vi "LINX - WS2812 Strip Controller.vi"() -> ()   [LabVIEW 2020]
doc: "Control the RGB colors of a WS2812 light strip using configurable sine, square, triangle and sawtooth waveforms for red, green and blue."
uses:
  vi.lib/MakerHub/LINX/Public/Utilities/Open Serial.vi
  vi.lib/MakerHub/LINX/Public/Sensors/Lights/WS2812/Write N LEDs.vi
  vi.lib/MakerHub/LINX/LMH-LINX.lvlib
  vi.lib/MakerHub/LINX/Public/Sensors/Lights/WS2812/WS2812.lvlib
panel:
  in  "Blue Duty Cycle":dbl=1.0 caption="Phase" min=0.0 max=100.0
  in  "Green Duty Cycle":dbl=1.0 caption="Phase" min=0.0 max=50.0
  in  "Red Duty Cycle":dbl=1.0 caption="Phase" min=0.0 max=100.0
  in  "Blue Waveform":enum16{"Sine", "Square", "Triangle", "Sawtooth"}(ring)
  in  "Green Waveform":enum16{"Sine", "Square", "Triangle", "Sawtooth"}(ring)
  in  "Red Waveform":enum16{"Sine", "Square", "Triangle", "Sawtooth"}(ring)
  in  "Blue Intensity Multiplier":dbl=1.0 caption="Phase" min=0.0 max=1.0
  in  "Green Intensity Multiplier":dbl=1.0 caption="Phase" min=0.0 max=1.0
  in  "Red Intensity Multiplier":dbl=1.0 caption="Phase" min=0.0 max=1.0
  in  "Blue Phase Multiplier":dbl=10.0 caption="Phase"
  in  "Blue Phase Offset":dbl=10.0 caption="Phase"
  in  "Green Phase Multiplier":dbl=10.0 caption="Phase"
  in  "Green Phase Offset":dbl=10.0 caption="Phase"
  in  "Red Phase Offset":dbl=10.0 caption="Phase"
  in  "Red Phase Multiplier":dbl=10.0 caption="Phase"
  out "RGB Values":dynamicdata(graph)
  in  "Stop Button":bool
  in  "Number of LEDs":u16=30
  in  "Data Channel":u8=11
  in  "Serial Port":refnum<visa-resource-name>="COM6"
  # "WS2812 Write N LEDs Example\n\nThis example demonstrates how to set the color of a range of WS2812 LEDs.\n\nInstructions\n1. Select the COM Port associated with the LINX Device.\n2. Select the Data Channel and Number of LEDs.\n3. Click the Run Arrow.\n4. Select the index of the first LED to set.\n5. The number values in the color array determines how many LEDs will be set, starting with the LED at the LED Start Index."
  # "LINX Device Settings"
  # "WS2812 Settings"
  # "Duty Cycle\n(Square Wave)"
  # "Intensity (0-1)"
  # "Phase Multiplier"
  # "Phase Offset"
  # "Waveform"
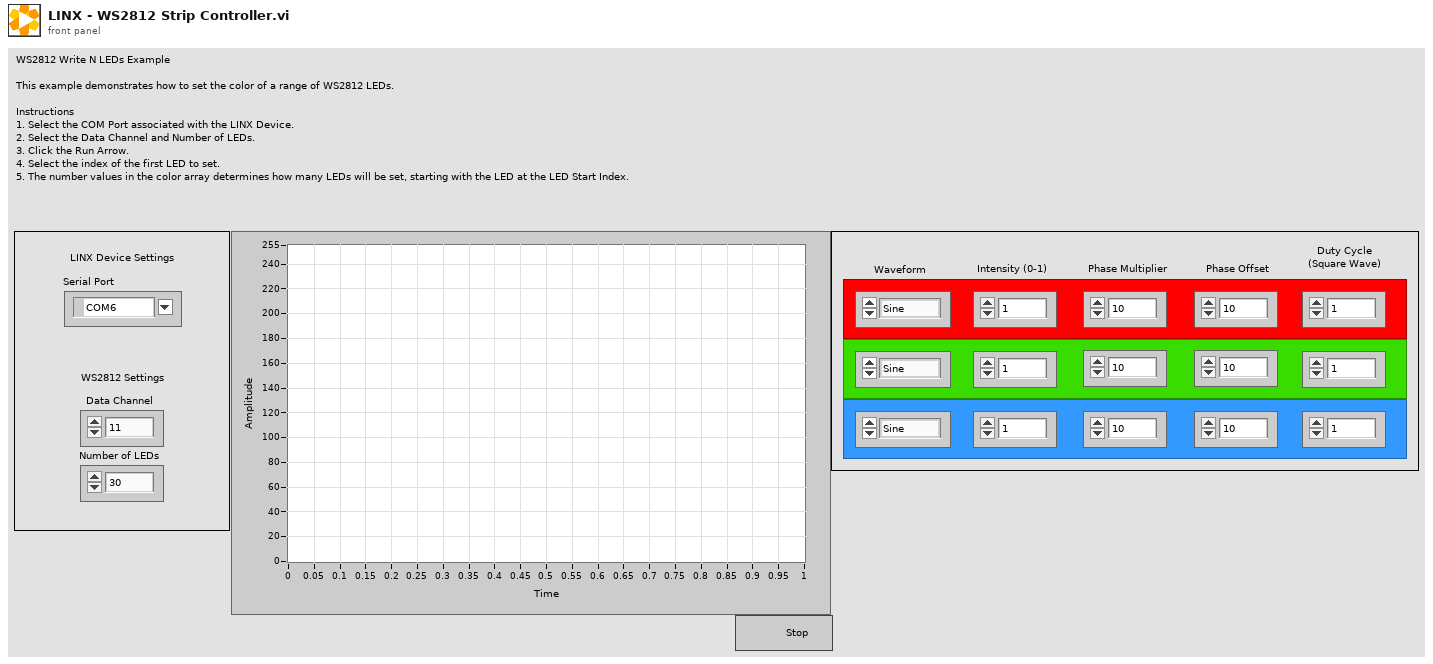
[diagram p1: front panel]
types:
  T1 = typedef "LMH-LINX.lvlib/LINX Ref.ctl" = cluster{"IO":T2, "Interface":T3, "LINX Device Config":T4}
  T2 = typedef "LMH-LINX.lvlib/Platform.ctl" = enum16{"Remote", "Local"}
  T3 = typedef "LMH-LINX.lvlib/Interface.ctl" = enum16{"Serial", "TCP"}
  T4 = typedef "Device.lvlib/LINX Device Config.ctl" = cluster{"Interface":T3, "COM Port":refnum<visa-resource-name>, "TCP Configuration":T5, "Device Family":u8, "Device ID":u8, "Device Name":string, "TCP Ref":refnum<k5>, "Channels":T6}
  T5 = typedef "Device.lvlib/TCP Config.ctl" = cluster{"IP Address":string, "Port":u16}
  T6 = typedef "LMH-LINX.lvlib/Channels.ctl" = cluster{"DI":u8[], "DO":u8[], "AI":u8[], "AO":u8[], "PWM":u8[], "QE":u8[], "UART":u8[], "I2C 2":u8[], "SPI":u8[], "CAN":u8[], "Servo":u8[], "AI Ref (V)":dbl, "AI Resolution (Bits)":u8, "AO Ref (V)":dbl, "AO Resolution (Bits)":u8}
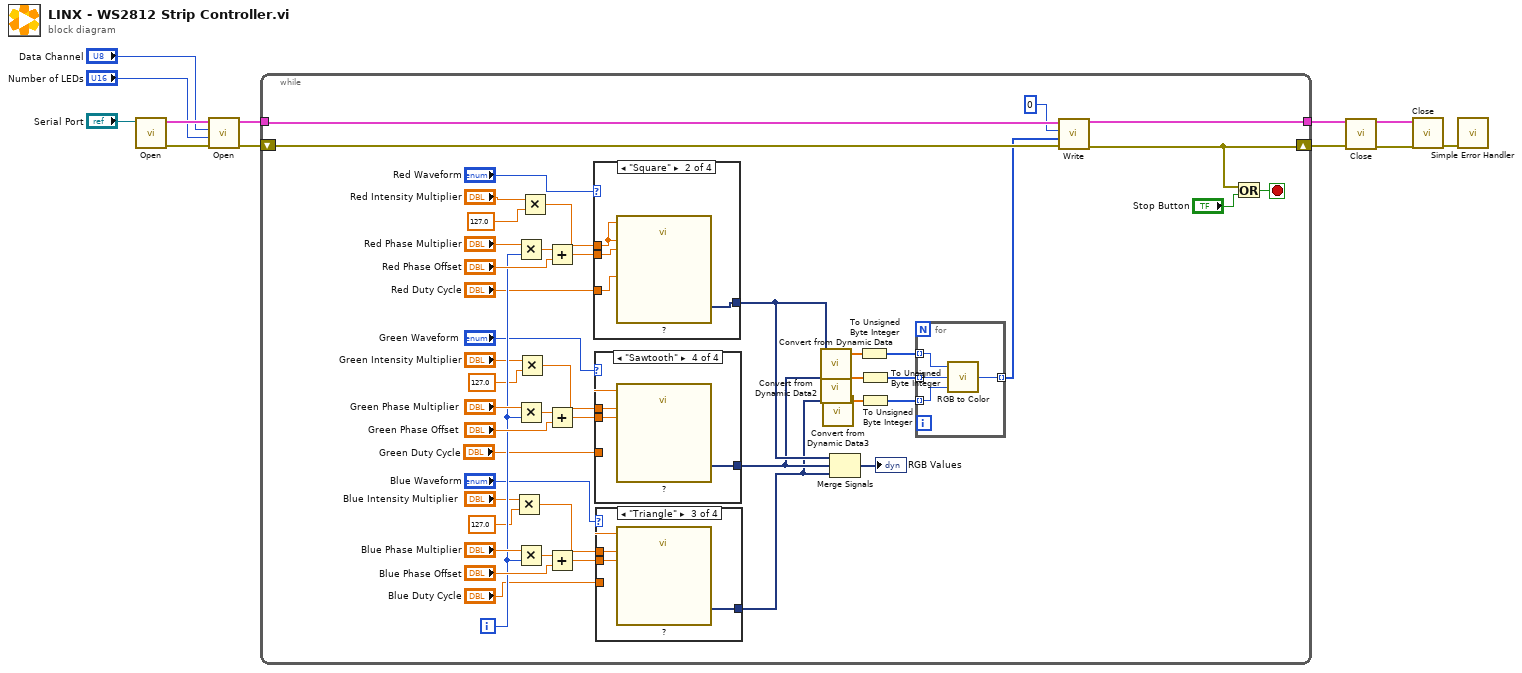
[diagram p0: block diagram]
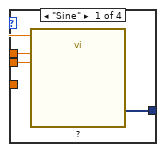
[diagram p2: hidden frame]
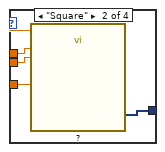
[diagram p3: hidden frame]
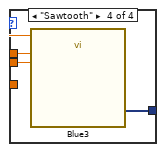
[diagram p4: hidden frame]
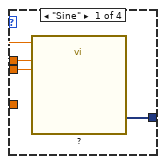
[diagram p5: hidden frame]
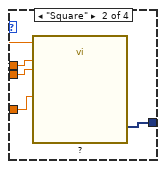
[diagram p6: hidden frame]
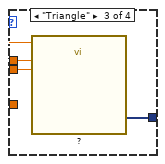
[diagram p7: hidden frame]
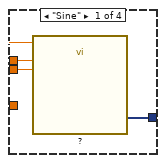
[diagram p8: hidden frame]
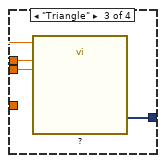
[diagram p9: hidden frame]
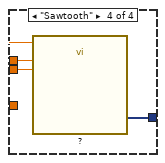
[diagram p10: hidden frame]
diagram:
  n1 = call-poly "Open.vi"("Serial Port"="Serial Port") -> ("Error Out"=w9:errorcluster, "LINX Resource"=w10:T1)  [unwired: 8 in, 1 out]
  n2 = call "Open.vi"("Error In"=w9, "Number of LEDs"="Number of LEDs", "Data Channel"="Data Channel", "LINX Resource"=w10) -> ("Error Out"=w8:errorcluster, "LINX Resource"=w7:T1)  [unwired: 6 in]
  n3 = while {
    tunnel: w7 -> [w56]
    shift-right: [w54] -> w4
    shift-left: w8 -> [w57]
    tunnel: [w55] -> w3
    i -> [w30]
    stop <- w58 stop-if-true
    n4 = Multiply(x="Blue Intensity Multiplier", y=127.0) -> (x*y=w20:dbl)
    n5 = Multiply(x="Red Phase Multiplier", y=w30) -> (x*y=w28:dbl)
    n6 = Multiply(x="Green Phase Multiplier", y=w30) -> (x*y=w48:dbl)
    n7 = Multiply(x="Blue Phase Multiplier", y=w30) -> (x*y=w45:dbl)
    n8 = Multiply(x="Green Intensity Multiplier", y=127.0) -> (x*y=w22:dbl)
    n9 = Multiply(x="Red Intensity Multiplier", y=127.0) -> (x*y=w21:dbl)
    n10 = Add(x=w28, y="Red Phase Offset") -> (x+y=w51:dbl)
    n11 = Add(x=w48, y="Green Phase Offset") -> (x+y=w50:dbl)
    n12 = Add(x=w45, y="Blue Phase Offset") -> (x+y=w43:dbl)
    n13 = case shown="\"Square\"" "Red Waveform" {
      tunnel: w51 -> [w87 w91 w94 w97]
      tunnel: [w86 w90 w93 w96] -> w36
      tunnel: w21 -> [w85 w89 w92 w95]
      tunnel: "Red Duty Cycle" -> [_ w88 _ _]
      frame "Sine" {
        n14 = call "?"("Offset"=w85, "Amplitude"=w85, "Phase"=w87) -> ("Red Sine"=w86:dynamicdata)  [unwired: 11 in, 1 out]
      }
      frame "Square" {
        n15 = call "?"("Offset"=w89, "Duty Cycle (%)"=w88, "Amplitude"=w89, "Phase"=w91) -> ("Red Square"=w90:dynamicdata)  [unwired: 10 in, 1 out]
      }
      frame "Triangle" {
        n16 = call "?"("Offset"=w92, "Amplitude"=w92, "Phase"=w94) -> ("Red Triangle"=w93:dynamicdata)  [unwired: 11 in, 1 out]
      }
      frame "Sawtooth" {
        n17 = call "?"("Offset"=w95, "Amplitude"=w95, "Phase"=w97) -> ("Red Sawtooth"=w96:dynamicdata)  [unwired: 11 in, 1 out]
      }
    }
    n18 = case shown="\"Sawtooth\"" "Green Waveform" {
      tunnel: w50 -> [w74 w78 w81 w84]
      tunnel: [w73 w77 w80 w83] -> w35
      tunnel: w22 -> [w72 w76 w79 w82]
      tunnel: "Green Duty Cycle" -> [_ w75 _ _]
      frame "Sine" {
        n19 = call "?"("Offset"=w72, "Amplitude"=w72, "Phase"=w74) -> ("Green Sine"=w73:dynamicdata)  [unwired: 11 in, 1 out]
      }
      frame "Square" {
        n20 = call "?"("Offset"=w76, "Duty Cycle (%)"=w75, "Amplitude"=w76, "Phase"=w78) -> ("Green Square"=w77:dynamicdata)  [unwired: 10 in, 1 out]
      }
      frame "Triangle" {
        n21 = call "?"("Offset"=w79, "Amplitude"=w79, "Phase"=w81) -> ("Green Triange"=w80:dynamicdata)  [unwired: 11 in, 1 out]
      }
      frame "Sawtooth" {
        n22 = call "?"("Offset"=w82, "Amplitude"=w82, "Phase"=w84) -> ("Green Sawtooth"=w83:dynamicdata)  [unwired: 11 in, 1 out]
      }
    }
    n23 = case shown="\"Triangle\"" "Blue Waveform" {
      tunnel: w43 -> [w61 w65 w68 w71]
      tunnel: [w60 w64 w67 w70] -> w34
      tunnel: w20 -> [w59 w63 w66 w69]
      tunnel: "Blue Duty Cycle" -> [_ w62 _ _]
      frame "Sine" {
        n24 = call "?"("Offset"=w59, "Amplitude"=w59, "Phase"=w61) -> ("Blue Sine"=w60:dynamicdata)  [unwired: 11 in, 1 out]
      }
      frame "Square" {
        n25 = call "?"("Offset"=w63, "Duty Cycle (%)"=w62, "Amplitude"=w63, "Phase"=w65) -> ("Blue Square"=w64:dynamicdata)  [unwired: 10 in, 1 out]
      }
      frame "Triangle" {
        n26 = call "?"("Offset"=w66, "Amplitude"=w66, "Phase"=w68) -> ("Blue Triangle"=w67:dynamicdata)  [unwired: 11 in, 1 out]
      }
      frame "Sawtooth" {
        n27 = call "Blue3"("Offset"=w69, "Amplitude"=w69, "Phase"=w71) -> ("Blue Sawtooth"=w70:dynamicdata)  [unwired: 11 in, 1 out]
      }
    }
    n28 = call "Convert from Dynamic Data"("Dynamic Data Type"=w36) -> ("Array"=w42:dbl[])  [unwired: 3 in]
    n29 = call "Convert from Dynamic Data2"("Dynamic Data Type"=w35) -> ("Array"=w40:dbl[])  [unwired: 3 in]
    n30 = call "Convert from Dynamic Data3"("Dynamic Data Type"=w34) -> ("Array"=w37:dbl[])  [unwired: 3 in]
    n31 = Merge Signals(w36, w35, w34) -> (→"RGB Values":dynamicdata)
    n32 = To Unsigned Byte Integer(number=w42) -> (unsigned 8bit integer=w41:u8[])
    n33 = To Unsigned Byte Integer(number=w40) -> (unsigned 8bit integer=w39:u8[])
    n34 = To Unsigned Byte Integer(number=w37) -> (unsigned 8bit integer=w38:u8[])
    n35 = for {
      tunnel: w41 -> [w101] mode=indexing
      tunnel: [w100] -> w33 mode=indexing
      tunnel: w39 -> [w99] mode=indexing
      tunnel: w38 -> [w98] mode=indexing
      n36 = call <vilib>:"RGB to Color.vi"("B"=w98, "G"=w99, "R"=w101) -> ("Color"=w100:u32)
    }
    n37 = call-poly "Write.vi"("Error In"=w57, "Colors"=w33, "LED Index"=u16 0, "LINX Ref"=w56) -> ("Error Out"=w54:errorcluster, "LINX Ref"=w55:T1)  [unwired: 6 in]
    n38 = Or(x=w54, y="Stop Button") -> (x .or. y?=w58:bool)
  }
  n39 = call "Close.vi"("Error In"=w4, "LINX Resource"=w3) -> ("Error Out"=w2:errorcluster, "LINX Resource"=w1:T1)  [unwired: 8 in]
  n40 = call "Close.vi"("Error In"=w2, "LINX Resource"=w1) -> ("Error Out"=w11:errorcluster)  [unwired: 9 in]
  n41 = call <vilib>:"Simple Error Handler.vi"("error in (no error)"=w11) -> ()  [unwired: 4 in, 5 out]
